vi "Read ILC Defaults.vi"(8 "error in (no error)":errorcluster, 11 "Boot Loader in":refnum<class "Boot Loader.lvclass">) -> (0 "error out":errorcluster, 2 "ILC Default Settings":T1 {"PGA Gain Coefficient" max=7}, 3 "Boot Loader out":refnum<class "Boot Loader.lvclass">)   [LabVIEW 2015, in "Boot Loader.lvclass"]
uses:
  Boot Loader.lvclass
  <userlib>/Common/ILC/Typedefs/ADC Settings.ctl
  <userlib>/Common/ILC/Configuration/Input Channels.ctl
  <userlib>/Common/ILC/Configuration/Scan Rates.ctl
  <userlib>/Common/ILC/Configuration/ILCConfiguration.lvlib
  <userlib>/Common/ILC/Typedefs/ILCTypedefs.lvlib
  Settings/Settings.lvclass
panel:
  # "Gain is 2^gain_coefficient"
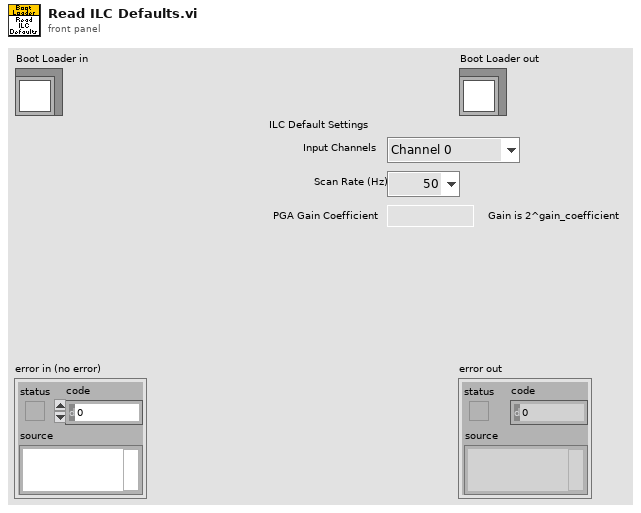
[diagram p1: front panel]
types:
  T1 = typedef "ILCCommon.lvlib/ILCTypedefs.lvlib/ADC Settings.ctl" = cluster{"Input Channels":T2, "Scan Rate (Hz) ":T3, "PGA Gain Coefficient":u8}
  T2 = typedef "ILCCommon.lvlib/ILCConfiguration.lvlib/Input Channels.ctl" = enum16{"Channel 0", "3 Channels", "5 Channels"}
  T3 = typedef "ILCCommon.lvlib/ILCConfiguration.lvlib/Scan Rates.ctl" = enum16{"50", "60", "100", "120", "200", "240", "300", "400", "480", "600", "1200", "2400", "4800"}
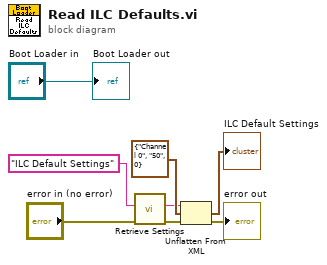
[diagram p0: block diagram]
diagram:
  n1 = call "Retrieve Settings.vi"("error in (no error)"="error in (no error)", "configName"="ILC Default Settings") -> ("error out"=w2:errorcluster, "xmlConfig"=w5:string)  [unwired: 7 in, 1 out]
  n2 = Unflatten From XML(xml string=w5, type=T1 {"Input Channels"=enum."Channel 0", "Scan Rate (Hz) "=enum."50", "PGA Gain Coefficient"=0} ("ADC Settings"), error in (no error)=w2) -> (value=→"ILC Default Settings":T1, error out=→"error out":errorcluster)
  "Boot Loader out" <- "Boot Loader in"
